vi "FlexDDS-NG_DCP_Sweep_down.vi"(4 "Step Size (Hz)":dbl, 5 "f1":dbl=30000000.0, 6 "jump before ramp":bool, 7 "f0":dbl=45000000.0, 8 "Ramp Rate":u16, 10 "Channels in":T1(ring), 11 "initial instruction string":string) -> (3 "appended instruction string out":string)   [LabVIEW 2016]
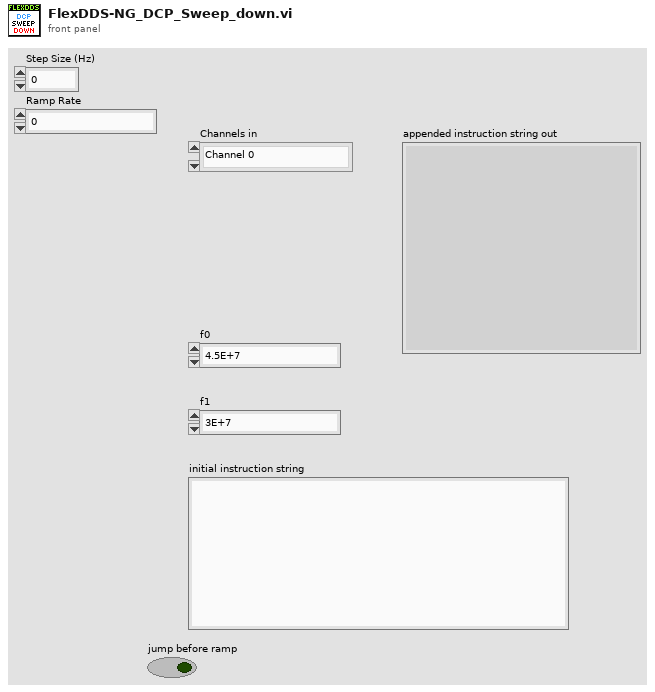
[diagram p1: front panel]
types:
  T1 = enum32{"Channel 0", "Channel 1", "Both channels"}
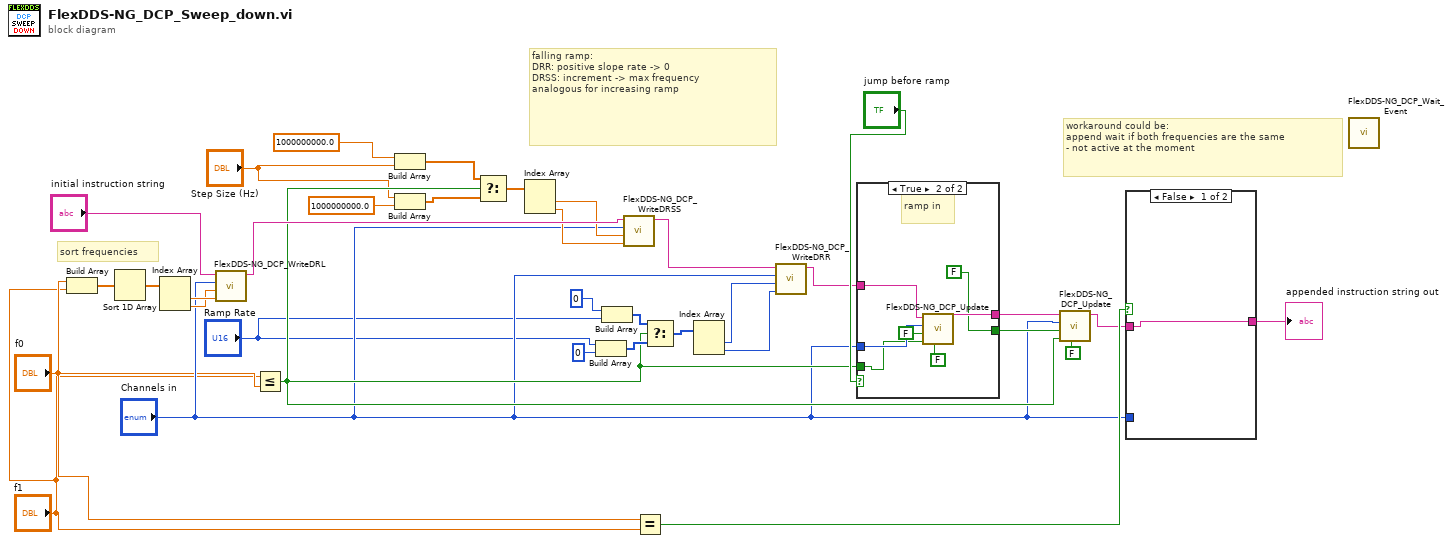
[diagram p0: block diagram]
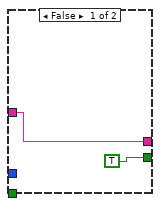
[diagram p3: hidden frame]
diagram:
  # "workaround could be:\nappend wait if both frequencies are the same\n- not active at the moment"
  # "falling ramp:\nDRR: positive slope rate -> 0\nDRSS: increment -> max frequency\nanalogous for increasing ramp"
  # "sort frequencies"
  n1 = Build Array("f0", "f1") -> (w31:dbl[])
  n2 = Sort 1D Array(array=w31) -> (sorted array=w32:dbl[])
  n3 = Index Array(array=w32) -> (element #1=w34:dbl, element #2=w33:dbl)  [unwired: 2 in]
  n4 = call "FlexDDS-NG_DCP_WriteDRL.vi"("low limit"=w34, "high limit"=w33, "Channels"="Channels in", "initial instruction string"="initial instruction string") -> ("appended instruction string"=w30:string)  [unwired: 7 in]
  n5 = Less Or Equal?(x="f1", y="f0") -> (x <= y?=w18:bool)
  n6 = Build Array(1000000000.0 ("element"), "Step Size (Hz)") -> (w15:dbl[])
  n7 = Build Array("Step Size (Hz)", 1000000000.0 ("element")) -> (w14:dbl[])
  n8 = Select(t=w15, s=w18, f=w14) -> (s? t:f=w13:dbl[])
  n9 = Index Array(array=w13) -> (element #1=w12:dbl, element #2=w11:dbl)  [unwired: 2 in]
  n10 = Build Array("Ramp Rate", u16 0 ("element")) -> (w28:u16[])
  n11 = Build Array(u16 0 ("element"), "Ramp Rate") -> (w27:u16[])
  n12 = call "FlexDDS-NG_DCP_WriteDRSS.vi"("increment step size"=w11, "decrement step size"=w12, "Channels"="Channels in", "initial instruction string"=w30) -> ("appended instruction string"=w29:string)  [unwired: 7 in]
  n13 = Equal?(x="f0", y="f1") -> (x = y?=w8:bool)
  n14 = Select(t=w27, s=w18, f=w28) -> (s? t:f=w26:u16[])
  n15 = Index Array(array=w26) -> (element #1=w25:u16, element #2=w24:u16)  [unwired: 2 in]
  n16 = call "FlexDDS-NG_DCP_WriteDRR.vi"("digital ramp positive slope rate"=w24, "digital ramp negative slope rate"=w25, "Channels"="Channels in", "initial instruction string"=w29) -> ("appended instruction string"=w22:string)  [unwired: 7 in]
  n17 = case shown="True" "jump before ramp" {
    tunnel: w22 -> [w37 w43]
    tunnel: [w37 w44] -> w21
    tunnel: "Channels in" -> [_ w42]
    tunnel: w18 -> [_ w38]
    tunnel: [TRUE FALSE ("IO_UPDATE(true=u, false = '')")] -> w9
    frame False {
    }
    frame True {
      # "ramp in"
      n18 = call "FlexDDS-NG_DCP_Update.vi"("ONLY IO_UPDATE"=FALSE, "DRCTL(true=+, false=-)"=w38, "IO_UPDATE(true=u, false = '')"=FALSE, "Channels"=w42, "appended instruction string in"=w43) -> ("appended instruction string out"=w44:string)  [unwired: 6 in]
    }
  }
  n19 = call "FlexDDS-NG_DCP_Update.vi"("ONLY IO_UPDATE"=FALSE, "DRCTL(true=+, false=-)"=w18, "IO_UPDATE(true=u, false = '')"=w9, "Channels"="Channels in", "appended instruction string in"=w21) -> ("appended instruction string out"=w7:string)  [unwired: 6 in]
  n20 = case shown="False" w8 {
    tunnel: w7 -> [w45 w46]
    tunnel: [w45 w46] -> w6
    tunnel: "Channels in" -> [_ _]
    frame False {
    }
    frame True {
    }
  }
  "appended instruction string out" <- w6
  n21 = call "FlexDDS-NG_DCP_Wait_Event.vi"() -> ()  [unwired: 11 in, 1 out]
